vi "destroy.vi"(8 "error in (no error)":errorcluster, 11 "llm_ollama_embedding in":refnum<class "llm_ollama_embedding.lvclass">) -> (0 "error out":errorcluster, 3 "llm_ollama_embedding out":refnum<class "llm_ollama_embedding.lvclass">)   [LabVIEW 2020, in "llm_ollama_embedding.lvclass"]
uses:
  llm_ollama_embedding.lvclass
  abstract_llm_base/abstract_llm_base.lvclass
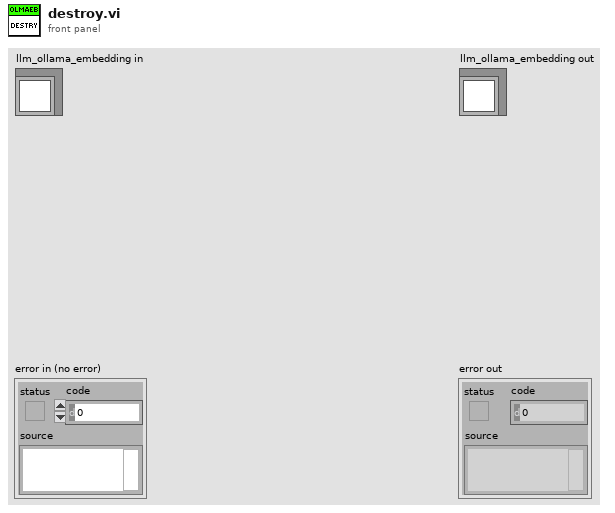
[diagram p1: front panel]
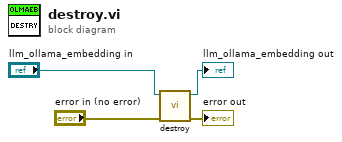
[diagram p0: block diagram]
diagram:
  n1 = call-parent "destroy.vi"("error in (no error)"="error in (no error)", "abstract_llm_base in"="llm_ollama_embedding in") -> ("error out"=→"error out":errorcluster, "abstract_llm_base out"=→"llm_ollama_embedding out":refnum<class "llm_ollama_embedding.lvclass">)  [unwired: 8 in]
